vi "Initialize DI.vi"(8 "error in (no error)":errorcluster, 9 "DI Channel Setting":T1, 10 "DAQ Type":enum16{"Hardware", "Simulation"}(ring), 11 "PXIe 6363 in":refnum<class "PXIe 6363.lvclass">) -> (0 "error out":errorcluster, 3 "PXIe 6363 out":refnum<class "PXIe 6363.lvclass">)   [LabVIEW 2021, in "DAQ Hardware.lvlib" / "PXIe 6363.lvclass"]
uses:
  PXIe 6363.lvclass
  DI Channel Setting.ctl
  PXIe 6363.lvclass/PXIe 6363.ctl
  DAQ Hardware.lvlib
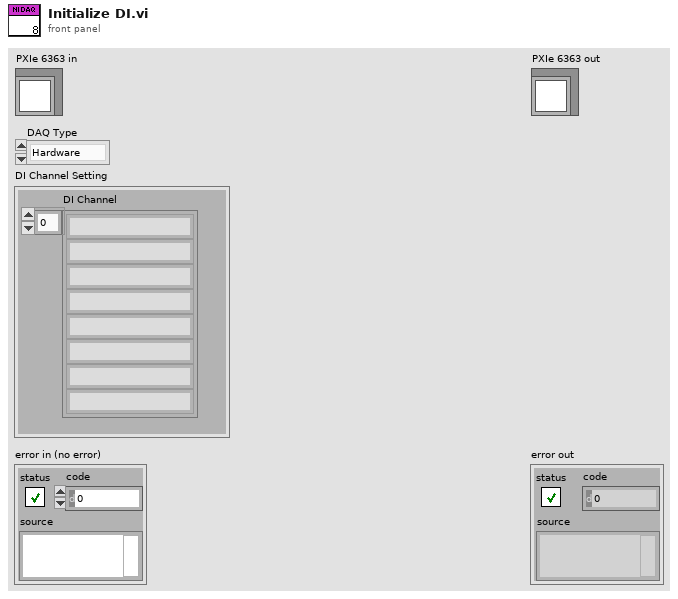
[diagram p1: front panel]
types:
  T1 = typedef "DAQ Hardware.lvlib/DI Channel Setting.ctl" = cluster{"DI Channel":string[]}
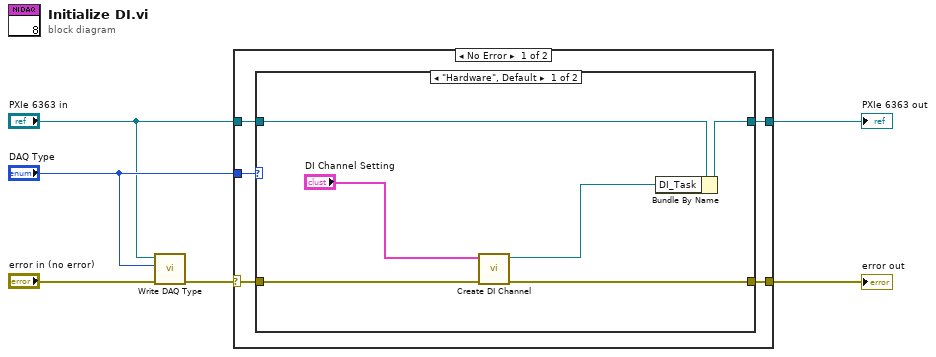
[diagram p0: block diagram]
diagram:
  n1 = call-dynamic "Write DAQ Type.vi"("error in (no error)"="error in (no error)", "DAQ Type"="DAQ Type", "PXIe 6363 in"="PXIe 6363 in") -> ("error out"=w5:errorcluster)  [unwired: 7 in, 1 out]
  n2 = case shown="No Error" w5 {
    selector: w5 -> [w11 w20]
    tunnel: "DAQ Type" -> [w10 _]
    tunnel: "PXIe 6363 in" -> [w9 w21]
    tunnel: [w8 w21] -> w2
    tunnel: [w7 w20] -> w1
    frame No Error {
      n3 = case shown="\"Hardware\", Default" w10 {
        tunnel: w11 -> [w17 w18]
        tunnel: w9 -> [w16 w19]
        tunnel: [w15 w19] -> w8
        tunnel: [w12 w18] -> w7
        frame "Hardware", Default {
          n4 = call "Create DI Channel.vi"("error in (no error)"=w17, "DI Channel Setting"="DI Channel Setting") -> ("error out"=w12:errorcluster, "DI_Task"=w14:refnum<k21>)  [unwired: 8 in]
          n5 = Bundle By Name(cluster=w16, "DI_Task"=w14) -> (w15:refnum<class "PXIe 6363.lvclass">)
        }
        frame "Simulation" {
        }
      }
    }
    frame Error {
    }
  }
  "error out" <- w1
  "PXIe 6363 out" <- w2
